vi "GetWriteVITemplatePath.vi"(7 "Include error terminals":bool, 8 "error in (no error)":errorcluster, 11 "ArrayElementScripter in":refnum<class "ArrayElementScripter.lvclass">) -> (0 "error out":errorcluster, 2 "VI Path":path, 3 "ArrayElementScripter out":refnum<class "ArrayElementScripter.lvclass">)   [LabVIEW 2021, in "MemberVICreation.lvlib" / "ArrayElementScripter.lvclass"]
uses:
  <resource>/Framework/Providers/LVClassLibrary/NewAccessors/ArrayElementScripter/ArrayElementScripter.lvclass
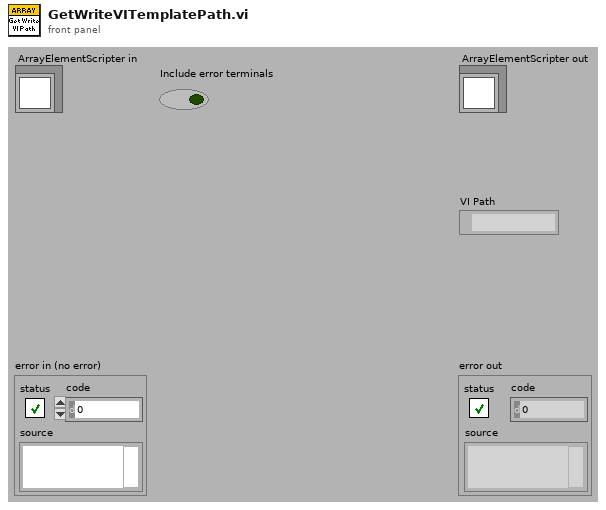
[diagram p1: front panel]
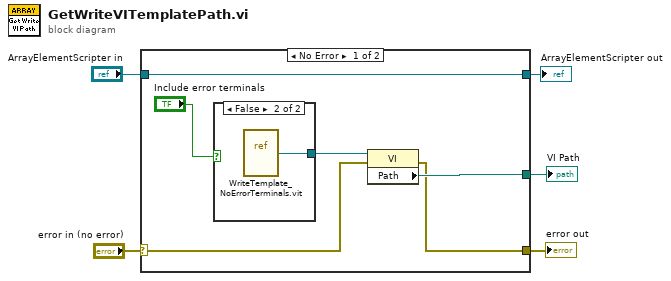
[diagram p0: block diagram]
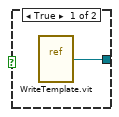
[diagram p2: hidden frame]
diagram:
  n1 = case shown="No Error" "error in (no error)" {
    selector: "error in (no error)" -> [w9 w15]
    tunnel: [w8 w15] -> w2
    tunnel: [w10 _] -> w1
    tunnel: "ArrayElementScripter in" -> [w7 w14]
    tunnel: [w7 w14] -> w3
    frame No Error {
      n2 = case shown="False" "Include error terminals" {
        tunnel: [w12 w13] -> w11
        frame True {
          n3 = vi-ref <resource>:"WriteTemplate.vit"() -> (w12:refnum<vi>)
        }
        frame False {
          n4 = vi-ref <resource>:"WriteTemplate_NoErrorTerminals.vit"() -> (w13:refnum<vi>)
        }
      }
      n5 = property class="VI"(reference=w11, error in=w9) -> (error out=w8:errorcluster, "Path"=w10:path)  [unwired: 1 out]
    }
    frame Error {
    }
  }
  "error out" <- w2
  "VI Path" <- w1
  "ArrayElementScripter out" <- w3
